vi "Process IMU readings.vi"(8 "Sensor Data in":u16[](array[numeric]), 11 "error in (no error)":errorcluster) -> (0 "error out":errorcluster, 2 "Gyro deg/s":cluster{dbl, dbl, dbl}, 3 "Accel g's":cluster{dbl, dbl, dbl}, 4 "Accel g's":dbl[](array[numeric]), 6 "Gyro deg/s":dbl[](array[numeric]))   [LabVIEW 2016]
panel:
  in  "Gyro s":dbl=16.4 format="%#_13g"
  in  "Acc s":dbl=2048.0 format="%#_13g"
  in  "Cluster":T1
  out "Gyro cluster":cluster{dbl, dbl, dbl}
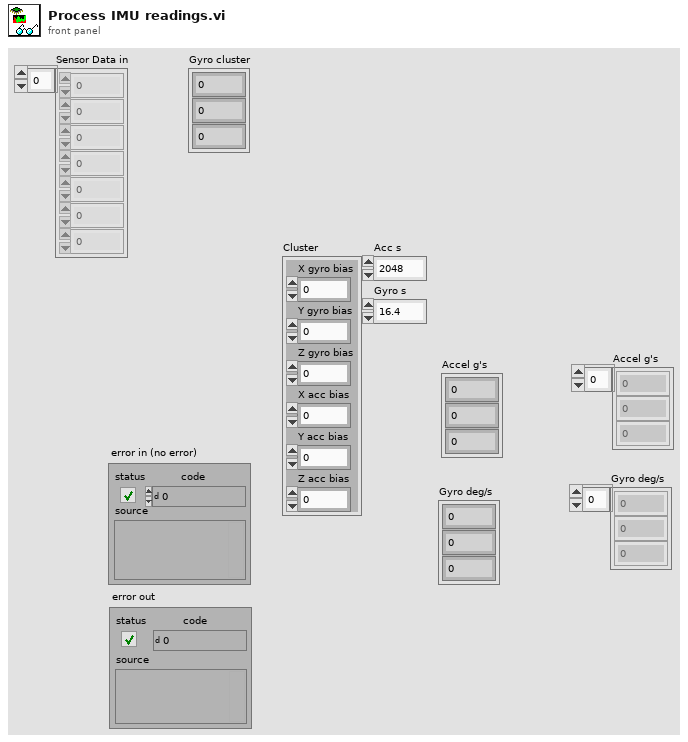
[diagram p1: front panel]
types:
  T1 = cluster{"X gyro bias":dbl, "Y gyro bias":dbl, "Z gyro bias":dbl, "X acc bias":dbl, "Y acc bias":dbl, "Z acc bias":dbl}
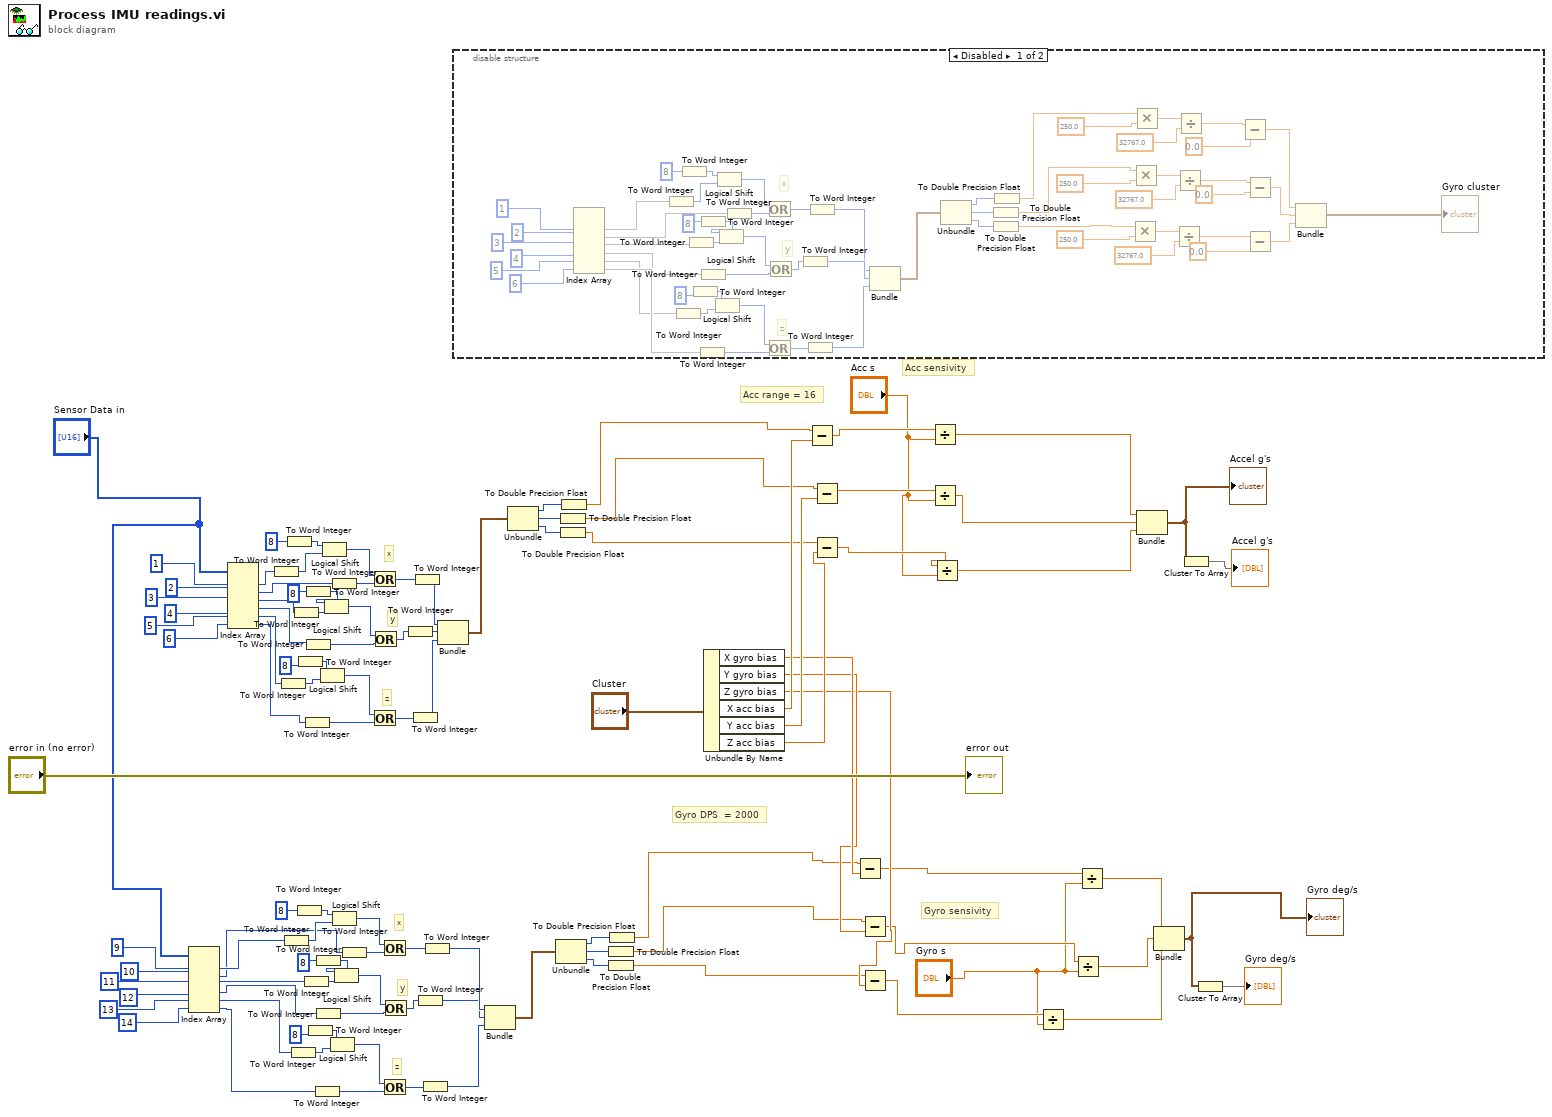
[diagram p0: block diagram]
diagram:
  # "Gyro sensivity"
  # "Acc sensivity"
  # "Acc range = 16"
  # "Gyro DPS  = 2000"
  # "z"
  # "y"
  # "x"
  # "z"
  # "y"
  # "x"
  n1 = Index Array(array="Sensor Data in", index #1=9 ("index"), index #2=10 ("index"), index #3=11 ("index"), index #4=12 ("index"), index #5=13 ("index"), index #6=14 ("index")) -> (element #1=w41:u16, element #2=w40:u16, element #3=w39:u16, element #4=w38:u16, element #5=w37:u16, element #6=w36:u16)
  n2 = Index Array(array="Sensor Data in", index #1=1 ("index"), index #2=2 ("index"), index #3=3 ("index"), index #4=4 ("index"), index #5=5 ("index"), index #6=6 ("index")) -> (element #1=w84:u16, element #2=w79:u16, element #3=w71:u16, element #4=w67:u16, element #5=w62:u16, element #6=w61:u16)
  n3 = To Word Integer(number=w84) -> (16bit integer=w83:i16)
  n4 = To Word Integer(number=w62) -> (16bit integer=w63:i16)
  n5 = To Word Integer(number=w41) -> (16bit integer=w48:i16)
  n6 = To Word Integer(number=i16 8 ("y")) -> (16bit integer=w82:i16)
  n7 = To Word Integer(number=w37) -> (16bit integer=w58:i16)
  n8 = To Word Integer(number=w71) -> (16bit integer=w68:i16)
  n9 = To Word Integer(number=i16 8 ("y")) -> (16bit integer=w49:i16)
  n10 = To Word Integer(number=i16 8 ("y")) -> (16bit integer=w64:i16)
  n11 = To Word Integer(number=w39) -> (16bit integer=w54:i16)
  n12 = To Word Integer(number=w61) -> (16bit integer=w60:i16)
  n13 = To Word Integer(number=i16 8 ("y")) -> (16bit integer=w69:i16)
  n14 = To Word Integer(number=w67) -> (16bit integer=w66:i16)
  n15 = To Word Integer(number=i16 8 ("y")) -> (16bit integer=w57:i16)
  n16 = To Word Integer(number=w36) -> (16bit integer=w59:i16)
  n17 = To Word Integer(number=i16 8 ("y")) -> (16bit integer=w53:i16)
  n18 = To Word Integer(number=w38) -> (16bit integer=w55:i16)
  n19 = Logical Shift(y=w64, x=w63) -> (x << y=w99:i16)
  n20 = Logical Shift(y=w82, x=w83) -> (x << y=w101:i16)
  n21 = Logical Shift(y=w69, x=w68) -> (x << y=w100:i16)
  n22 = Logical Shift(y=w57, x=w58) -> (x << y=w44:i16)
  n23 = To Word Integer(number=w79) -> (16bit integer=w80:i16)
  n24 = Logical Shift(y=w49, x=w48) -> (x << y=w42:i16)
  n25 = Logical Shift(y=w53, x=w54) -> (x << y=w43:i16)
  n26 = To Word Integer(number=w40) -> (16bit integer=w51:i16)
  n27 = Or(x=w101, y=w80) -> (x .or. y?=w90:i16)
  n28 = Or(x=w99, y=w60) -> (x .or. y?=w87:i16)
  n29 = Or(x=w100, y=w66) -> (x .or. y?=w86:i16)
  n30 = Or(x=w42, y=w51) -> (x .or. y?=w45:i16)
  n31 = Or(x=w44, y=w59) -> (x .or. y?=w46:i16)
  n32 = Or(x=w43, y=w55) -> (x .or. y?=w47:i16)
  n33 = To Word Integer(number=w86) -> (16bit integer=w88:i16)
  n34 = To Word Integer(number=w87) -> (16bit integer=w85:i16)
  n35 = To Word Integer(number=w90) -> (16bit integer=w89:i16)
  n36 = To Word Integer(number=w47) -> (16bit integer=w34:i16)
  n37 = To Word Integer(number=w46) -> (16bit integer=w33:i16)
  n38 = To Word Integer(number=w45) -> (16bit integer=w35:i16)
  n39 = Bundle(w89, w88, w85) -> (w91:cluster{i16, i16, i16})  [unwired: 1 in]
  n40 = disable-structure shown="Disabled" {
    frame Disabled {
      # "z"
      # "y"
      # "x"
      n41 = Index Array(index #1=1 ("index"), index #2=2 ("index"), index #3=3 ("index"), index #4=4 ("index"), index #5=5 ("index"), index #6=6 ("index")) -> (array=w166:u16[], element #1=w157, element #2=w158, element #3=w159, element #4=w160, element #5=w161, element #6=w162)
      n42 = To Word Integer(number=w157) -> (16bit integer=w150:i16)
      n43 = To Word Integer(number=w161) -> (16bit integer=w140:i16)
      n44 = To Word Integer(number=i16 8 ("y")) -> (16bit integer=w149:i16)
      n45 = To Word Integer(number=w159) -> (16bit integer=w144:i16)
      n46 = To Word Integer(number=i16 8 ("y")) -> (16bit integer=w141:i16)
      n47 = To Word Integer(number=w162) -> (16bit integer=w139:i16)
      n48 = To Word Integer(number=i16 8 ("y")) -> (16bit integer=w145:i16)
      n49 = To Word Integer(number=w160) -> (16bit integer=w143:i16)
      n50 = Logical Shift(y=w141, x=w140) -> (x << y=w154:i16)
      n51 = Logical Shift(y=w149, x=w150) -> (x << y=w156:i16)
      n52 = Logical Shift(y=w145, x=w144) -> (x << y=w155:i16)
      n53 = To Word Integer(number=w158) -> (16bit integer=w147:i16)
      n54 = Or(x=w156, y=w147) -> (x .or. y?=w153:i16)
      n55 = Or(x=w154, y=w139) -> (x .or. y?=w152:i16)
      n56 = Or(x=w155, y=w143) -> (x .or. y?=w151:i16)
      n57 = To Word Integer(number=w151) -> (16bit integer=w164:i16)
      n58 = To Word Integer(number=w152) -> (16bit integer=w165:i16)
      n59 = To Word Integer(number=w153) -> (16bit integer=w163:i16)
      n60 = Bundle(w163, w164, w165) -> (w138:cluster{i16, i16, i16})  [unwired: 1 in]
      n61 = Unbundle(w138) -> (w136:i16, w134:i16, w133:i16)
      n62 = To Double Precision Float(number=w134) -> (double precision float=w124:dbl)
      n63 = To Double Precision Float(number=w133) -> (double precision float=w123:dbl)
      n64 = To Double Precision Float(number=w136) -> (double precision float=w135:dbl)
      n65 = Multiply(x=w123, y=250.0) -> (x*y=w127:dbl)
      n66 = Multiply(x=w124, y=250.0) -> (x*y=w128:dbl)
      n67 = Multiply(x=w135, y=250.0) -> (x*y=w137:dbl)
      n68 = Divide(x=w127, y=32767.0) -> (x/y=w115:dbl)
      n69 = Divide(x=w128, y=32767.0) -> (x/y=w116:dbl)
      n70 = Divide(x=w137, y=32767.0) -> (x/y=w122:dbl)
      n71 = Subtract(x=w122, y=0.0) -> (x-y=w120:dbl)
      n72 = Subtract(x=w116, y=0.0) -> (x-y=w114:dbl)
      n73 = Subtract(x=w115, y=0.0) -> (x-y=w117:dbl)
      n74 = Bundle(w120, w114, w117) -> (→"Gyro cluster":cluster{dbl, dbl, dbl})  [unwired: 1 in]
    }
    frame Enabled {
    }
  }
  n75 = Bundle(w35, w34, w33) -> (w72:cluster{i16, i16, i16})  [unwired: 1 in]
  n76 = Unbundle(w91) -> (w78:i16, w77:i16, w76:i16)
  n77 = Unbundle(w72) -> (w73:i16, w74:i16, w75:i16)
  n78 = To Double Precision Float(number=w77) -> (double precision float=w6:dbl)
  n79 = To Double Precision Float(number=w76) -> (double precision float=w5:dbl)
  n80 = To Double Precision Float(number=w78) -> (double precision float=w7:dbl)
  n81 = To Double Precision Float(number=w74) -> (double precision float=w3:dbl)
  n82 = To Double Precision Float(number=w75) -> (double precision float=w2:dbl)
  n83 = To Double Precision Float(number=w73) -> (double precision float=w4:dbl)
  n84 = Unbundle By Name("Cluster") -> ("X gyro bias"=w26:dbl, "Y gyro bias"=w25:dbl, "Z gyro bias"=w24:dbl, "X acc bias"=w29:dbl, "Y acc bias"=w28:dbl, "Z acc bias"=w27:dbl)
  n85 = Subtract(x=w7, y=w29) -> (x-y=w17:dbl)
  n86 = Subtract(x=w6, y=w28) -> (x-y=w18:dbl)
  n87 = Subtract(x=w5, y=w27) -> (x-y=w19:dbl)
  n88 = Subtract(x=w4, y=w26) -> (x-y=w23:dbl)
  n89 = Subtract(x=w3, y=w25) -> (x-y=w21:dbl)
  n90 = Subtract(x=w2, y=w24) -> (x-y=w13:dbl)
  n91 = Divide(x=w17, y="Acc s") -> (x/y=w16:dbl)
  n92 = Divide(x=w18, y="Acc s") -> (x/y=w15:dbl)
  n93 = Divide(x=w19, y="Acc s") -> (x/y=w14:dbl)
  n94 = Divide(x=w13, y="Gyro s") -> (x/y=w12:dbl)
  n95 = Divide(x=w21, y="Gyro s") -> (x/y=w20:dbl)
  n96 = Divide(x=w23, y="Gyro s") -> (x/y=w22:dbl)
  n97 = Bundle(w16, w15, w14) -> (w10:cluster{dbl, dbl, dbl})  [unwired: 1 in]
  "Accel g's" <- w10
  n98 = Bundle(w22, w20, w12) -> (w31:cluster{dbl, dbl, dbl})  [unwired: 1 in]
  "Gyro deg/s" <- w31
  n99 = Cluster To Array(cluster=w10) -> (array=→"Accel g's":dbl[])
  n100 = Cluster To Array(cluster=w31) -> (array=→"Gyro deg/s":dbl[])
  "error out" <- "error in (no error)"
